vi "Combine Functions and Controls in a Palette File.vi"() -> ()   [LabVIEW 2023]
doc: "This VI shows how to create a single .mnu file that provides subpalettes in both the Controls and Functions palettes."
uses:
  <vilib>/Palette API/Palette Menu/Public Type Define/Palette type.ctl
  <vilib>/Palette API/Palette Menu/Public Type Define/Item.ctl
  <vilib>/Palette API/Palette Menu/Public Type Define/Palette Data.ctl
  <vilib>/Palette API/Palette Menu/Public Type Define/View Format.ctl
  <vilib>/Palette API/Palette Menu/Public Type Define/Items.ctl
  <vilib>/Palette API/Palette Menu/Public Type Define/Help Info.ctl
  <vilib>/Palette API/Palette Menu/Public Type Define/Synchronize Info.ctl
  <vilib>/Palette API/Palette Menu/Palette Menu.lvlib
panel:
  in  "display name (controls)":string="Sample Controls Palette"
  in  "display name (functions)":string="Sample Functions Palette"
  # "Overview: Demonstrates the use of the Palette Editing VIs to create a new palette file that contains contents for both the Controls and the Functions palettes.\nInstructions:\nRun the VI. You will now have new Functions > User Libraries > Sample Functions Palette and Controls > User Controls > Sample Controls Palette subpalettes. See the block diagram for more information.\n\nNote: To remove this new subpalette, delete the following file and restart LabVIEW: [LabVIEW]\\user.lib\\sample.mnu"
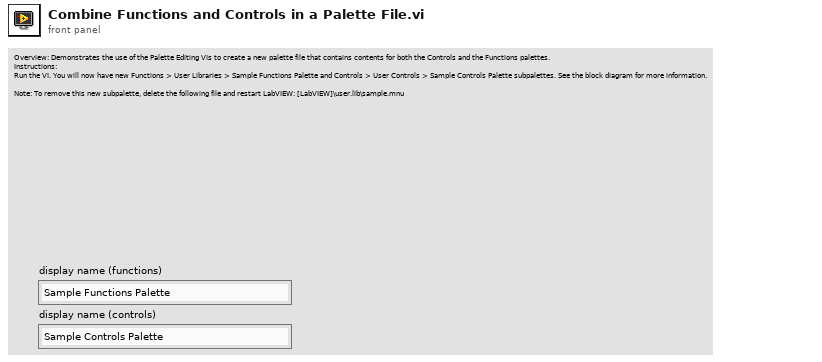
[diagram p1: front panel]
types:
  T1 = typedef "Palette Menu.lvlib/Palette Data.ctl" = cluster{"display name":string, "view format":T2, "palette width":i16, "items":T3, "256 color icon":picture, "B&W color icon":picture, "help information":T5, "palette description":string, "synchronize information":T6}
  T2 = typedef "Palette Menu.lvlib/View Format.ctl" = u16
  T3 = typedef "Palette Menu.lvlib/Items.ctl" = T4[]
  T4 = typedef "Palette Menu.lvlib/Item.ctl" = cluster{"item path":path, "library path":path, "use default lvlib palette":bool, "short name":string, "place VI contents":bool, "hide synchronized item":bool, "reserve spot for synch item":bool, "configure when placing VI contents":bool}
  T5 = typedef "Palette Menu.lvlib/Help Info.ctl" = cluster{"help tag":string, "help file path ":path}
  T6 = typedef "Palette Menu.lvlib/Synchronize Info.ctl" = cluster{"synchronize with directory":bool, "synchronize directory path":path}
  T7 = typedef "Palette Menu.lvlib/Palette type.ctl" = i32
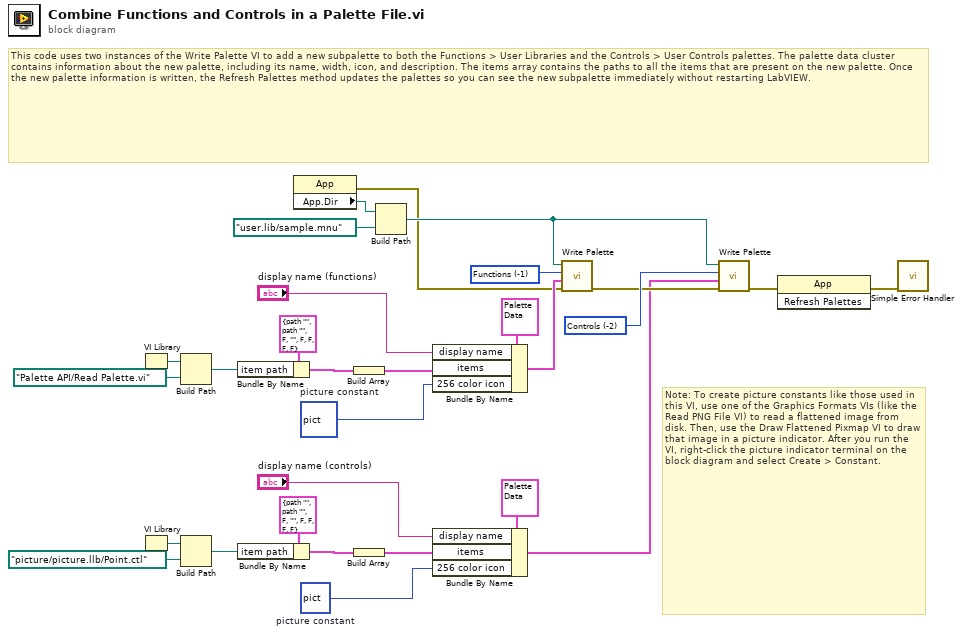
[diagram p0: block diagram]
diagram:
  w10 = picture bytes[3230]  # picture constant
  w11 = picture bytes[1246]  # picture constant
  w28 = T7 -2 items=["Functions"=-1, "Controls"=-2] ("palette type")
  w29 = T7 -1 items=["Functions"=-1, "Controls"=-2] ("palette type")
  # "Note: To create picture constants like those used in this VI, use one of the Graphics Formats VIs (like the Read PNG File VI) to read a flattened image from disk. Then, use the Draw Flattened Pixmap VI to draw that image in a picture indicator. After you run the VI, right-click the picture indicator terminal on the block diagram and select Create > Constant."
  # "This code uses two instances of the Write Palette VI to add a new subpalette to both the Functions > User Libraries and the Controls > User Controls palettes. The palette data cluster contains information about the new palette, including its name, width, icon, and description. The items array contains the paths to all the items that are present on the new palette. Once the new palette information is written, the Refresh Palettes method updates the palettes so you can see the new subpalette immediately without restarting LabVIEW."
  n1 = VI Library() -> (path=w8:path)
  n2 = VI Library() -> (path=w18:path)
  n3 = Build Path(base path=w8, name or relative path=path "Palette API/Read Palette.vi") -> (appended path=w6:path)
  n4 = Build Path(base path=w18, name or relative path=path "picture/picture.llb/Point.ctl") -> (appended path=w16:path)
  n5 = Bundle By Name(cluster=T4 {"item path"=path "", "library path"=path "", "use default lvlib palette"=FALSE, "short name"="", "place VI contents"=FALSE, "hide synchronized item"=FALSE, "reserve spot for synch item"=FALSE, "configure when placing VI contents"=FALSE} ("Items"), "item path"=w6) -> (w23:T4)
  n6 = Bundle By Name(cluster=T4 {"item path"=path "", "library path"=path "", "use default lvlib palette"=FALSE, "short name"="", "place VI contents"=FALSE, "hide synchronized item"=FALSE, "reserve spot for synch item"=FALSE, "configure when placing VI contents"=FALSE} ("Items"), "item path"=w16) -> (w20:T4)
  n7 = property class="App"() -> (error out=w1:errorcluster, "App.Dir"=w9:path)  [unwired: 2 in, 1 out]
  n8 = Build Array(w23) -> (w22:T4[])
  n9 = Build Array(w20) -> (w19:T4[])
  n10 = Build Path(base path=w9, name or relative path=path "user.lib/sample.mnu") -> (appended path=w12:path)
  n11 = Bundle By Name(cluster=T1 {"display name"="", "view format"=0, "palette width"=4, "items"=[], "256 color icon"=bytes[0], "B&W color icon"=bytes[0], "help information"={"help tag"="", "help file path "=path ""}, "palette description"="", "synchronize information"={"synchronize with directory"=FALSE, "synchronize directory path"=path ""}} ("Palette  Data"), "display name"="display name (functions)", "items"=w22, "256 color icon"=w10) -> (w27:T1)
  n12 = Bundle By Name(cluster=T1 {"display name"="", "view format"=0, "palette width"=4, "items"=[], "256 color icon"=bytes[0], "B&W color icon"=bytes[0], "help information"={"help tag"="", "help file path "=path ""}, "palette description"="", "synchronize information"={"synchronize with directory"=FALSE, "synchronize directory path"=path ""}} ("Palette  Data"), "display name"="display name (controls)", "items"=w19, "256 color icon"=w11) -> (w25:T1)
  n13 = call <vilib>:"Write Palette.vi"("error in (no error)"=w1, "palette data"=w27, "palette type"=w29, "palette path"=w12) -> ("error out"=w26:errorcluster)  [unwired: 1 in, 6 out]
  n14 = call <vilib>:"Write Palette.vi"("error in (no error)"=w26, "palette data"=w25, "palette type"=w28, "palette path"=w12) -> ("error out"=w15:errorcluster)  [unwired: 1 in, 6 out]
  n15 = invoke class="App" method="Refresh Palettes"(error in=w15) -> (error out=w14:errorcluster)  [unwired: 2 in, 2 out]
  n16 = call <vilib>:"Simple Error Handler.vi"("error in (no error)"=w14) -> ()  [unwired: 1 in, 8 out]
